vi "Configure Instrument Mode.vi"(7 "Unit Address (1)":u8=1, 8 "error in (no error)":errorcluster, 10 "Instrument Mode (0: Normal)":u8(ring) items=["Normal", "StandBy", "Configuration"], 11 "VISA resource name":refnum<visa-resource-name>) -> (0 "error out":errorcluster, 3 "VISA resource name out":refnum<visa-resource-name>)   [LabVIEW 2014, in "Eurotherm 35xx Series.lvlib"]
doc: "This VI sets instrument mode.\n\nWarning: Change default value interrupt working process (device will not control).\nIt is recommended that the device be disconnected from any active process."
uses:
  <instrlib>/Eurotherm 35xx Series/Eurotherm 35xx Series.lvlib
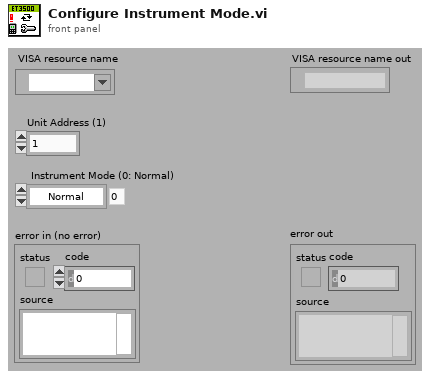
[diagram p1: front panel]
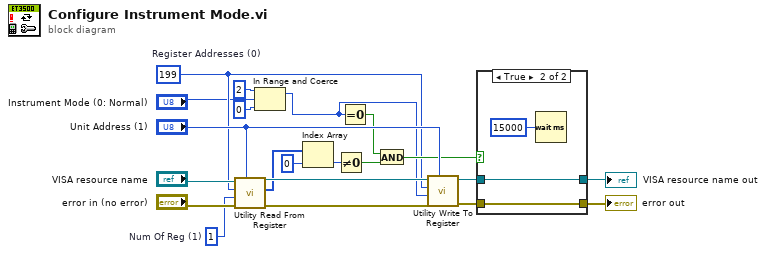
[diagram p0: block diagram]
diagram:
  w16 = u16 1  # Num Of Reg (1)
  w5 = 199  # Register Addresses (0)
  n1 = call <instrlib>:"Utility Read From Register.vi"("Unit Address (1)"="Unit Address (1)", "error in (no error)"="error in (no error)", "Num Of Reg (1)"=w16, "Register Address (0)"=w5, "VISA resource name"="VISA resource name") -> ("error out"=w20:errorcluster, "Data"=w15:i16[], "VISA resource name out"=w19:refnum<visa-resource-name>)  [unwired: 4 in]
  n2 = In Range and Coerce(upper limit=u8 2, x="Instrument Mode (0: Normal)", lower limit=u8 0) -> (coerced(x)=w3:u8)  [unwired: 1 out]
  n3 = Index Array(array=w15, index=0) -> (element=w13:i16)
  n4 = Not Equal To 0?(x=w13) -> (x != 0?=w12:bool)
  n5 = Equal To 0?(x=w3) -> (x = 0?=w11:bool)
  n6 = And(x=w11, y=w12) -> (x .and. y?=w6:bool)
  n7 = call <instrlib>:"Utility Write To Register.vi"("Unit Address (1)"="Unit Address (1)", "error in (no error)"=w20, "Data (0)"=w3, "Register Address (0)"=w5, "VISA resource name"=w19) -> ("error out"=w8:errorcluster, "VISA resource name out"=w10:refnum<visa-resource-name>)  [unwired: 5 in]
  n8 = case shown="True" w6 {
    tunnel: w10 -> [w23 w26]
    tunnel: [w23 w26] -> w9
    tunnel: w8 -> [w22 w25]
    tunnel: [w22 w25] -> w7
    frame False {
    }
    frame True {
      n9 = Wait (ms)(milliseconds to wait=u32 15000) -> ()  [unwired: 1 out]
    }
  }
  "error out" <- w7
  "VISA resource name out" <- w9
